vi "Stop Acquisition.vi"(8 "error in (no error)":T3 caption="entrée d'erreur (pas d'erreur)", 11 "Ressources matérielles en entrée":T1={"Refnum de matériel <À remplacer>"="", "Type de signal <À remplacer>"=enum."Sine Wave", "Choix de la longueur d'onde"=500.0, "Nom du périphérique"="Dev1", "Choix mode"=FALSE}) -> (0 "error out":T3 caption="sortie d'erreur")   [LabVIEW 2020, in "Acquisition.lvlib"]
doc: "Arrête l'acquisition."
uses:
  Acquisition.lvlib
  Hardware Configuration.ctl
  Signal Type.ctl
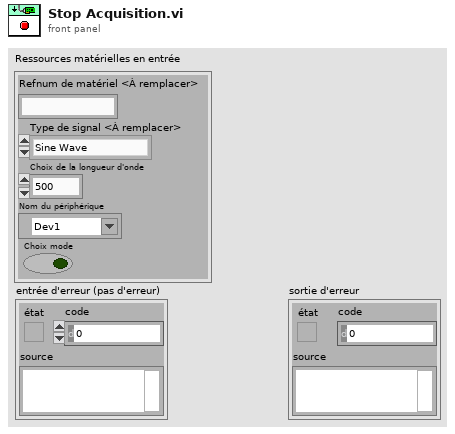
[diagram p1: front panel]
types:
  T1 = typedef "Acquisition.lvlib/Hardware Configuration.ctl" = cluster{"Refnum de matériel <À remplacer>":string, "Type de signal <À remplacer>":T2, "Choix de la longueur d'onde":dbl, "Nom du périphérique":tag, "Choix mode":bool}
  T2 = typedef "Acquisition.lvlib/Signal Type.ctl" = enum16{"Sine Wave", "Square with Noise", "Signal triangulaire", "Simulation DAQ"}
  T3 = cluster{"état":bool, "code":i32, "source":string}
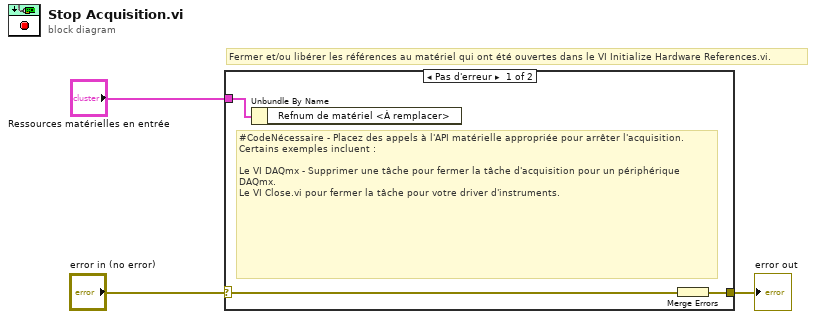
[diagram p0: block diagram]
diagram:
  # "Fermer et/ou libérer les références au matériel qui ont été ouvertes dans le VI Initialize Hardware References.vi."
  n1 = case shown="Pas d'erreur" "error in (no error)" {
    selector: "error in (no error)" -> [w5 w7]
    tunnel: [w6 w7] -> w2
    tunnel: "Ressources matérielles en entrée" -> [w4 _]
    frame No Error {
      # "#CodeNécessaire - Placez des appels à l'API matérielle appropriée pour arrêter l'acquisition.  Certains exemples incluent :\n\nLe VI DAQmx - Supprimer une tâche pour fermer la tâche d'acquisition pour un périphérique DAQmx.\nLe VI Close.vi pour fermer la tâche pour votre driver d'instruments."
      n2 = Unbundle By Name(w4) -> ()  [unwired: 1 out]
      n3 = Merge Errors(w5) -> (w6:errorcluster)
    }
    frame Error {
    }
  }
  "error out" <- w2
